vi "teleop2.vi"(7 "Control Type":enum32{"Logitech Joysticks", "Logitech Gamepad"}(ring), 8 "Match Info":T2={"Autonomous Elapsed Seconds"=0.0, "TeleOp Elapsed Seconds"=0.0, "Disabled Elapsed Seconds"=0.0, "Visited Autonomous"=FALSE, "Visited TeleOp"=FALSE, "Visited Disabled"=FALSE, "Autonomous Settings"={"Autonomous Style"=enum."Independent", "VI Refnum"=refnum}}, 11 "Call Context":T1) -> ()   [LabVIEW 2011]
uses:
  <vilib>/Rock Robotics/WPI/DriverStation/WPI_DriverStationMatch Info.ctl
  <vilib>/Rock Robotics/WPI/DriverStation/WPI_DriverStationDerivedRobotMode.ctl
  Robot Global Data.vi
  System Set Points and States.vi
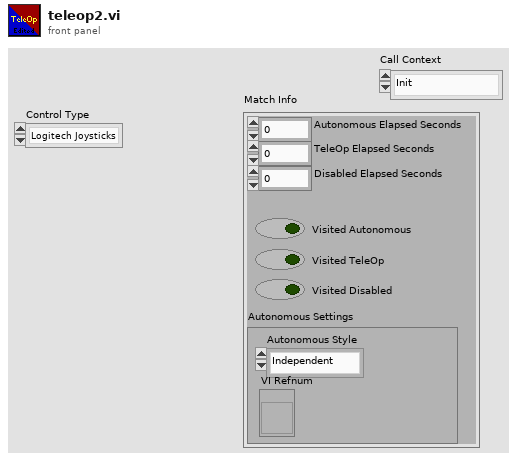
[diagram p1: front panel]
types:
  T1 = typedef "WPI_DriverStationDerivedRobotMode.ctl" = enum16{"Init", "Execute", "Stop"}
  T2 = typedef "WPI_DriverStationMatch Info.ctl" = cluster{"Autonomous Elapsed Seconds":dbl, "TeleOp Elapsed Seconds":dbl, "Disabled Elapsed Seconds":dbl, "Visited Autonomous":bool, "Visited TeleOp":bool, "Visited Disabled":bool, "Autonomous Settings":cluster{"Autonomous Style":enum16{"Iterative", "Independent"}, "VI Refnum":refnum<vi>}}
  T3 = cluster{"Position":cluster{"X":dbl, "Y":dbl}, "Distance (ft)":dbl}[]
  T4 = cluster{"Target Info[0]":cluster{"Position":cluster{"X":dbl, "Y":dbl}, "Distance (ft)":dbl}, "Target Info[1]":cluster{"Position":cluster{"X":dbl, "Y":dbl}, "Distance (ft)":dbl}, "Target Info[2]":cluster{"Position":cluster{"X":dbl, "Y":dbl}, "Distance (ft)":dbl}, "Target Info[3]":cluster{"Position":cluster{"X":dbl, "Y":dbl}, "Distance (ft)":dbl}, "Target Info[4]":cluster{"Position":cluster{"X":dbl, "Y":dbl}, "Distance (ft)":dbl}, "Target Info[5]":cluster{"Position":cluster{"X":dbl, "Y":dbl}, "Distance (ft)":dbl}, "Target Info[6]":cluster{"Position":cluster{"X":dbl, "Y":dbl}, "Distance (ft)":dbl}, "Target Info[7]":cluster{"Position":cluster{"X":dbl, "Y":dbl}, "Distance (ft)":dbl}, "Target Info[8]":cluster{"Position":cluster{"X":dbl, "Y":dbl}, "Distance (ft)":dbl}}
  T5 = typedef "WPI_MotorControlDeviceRef.ctl" = cluster{"DeviceStatus":errorcluster, "Type":enum16{"PWM", "CAN"}, "PWM":cluster{"Digital Module":T6, "PWM Channel":T7, "DeadBand":T8}, "CAN":cluster{"Device Number":u8, "Control Mode":T9, "Semaphore":T10, "Max Vout":dbl}, "Invert":bool, "TransformRef":T11, "InvTransformRef":T11}
  T6 = typedef "FPGA_TypedefDigitalModule.ctl" = enum16{"Digital Module 1", "Digital Module 2"}
  T7 = typedef "FPGA_DIOPWMChannel.ctl" = enum8{"PWM 1", "PWM 2", "PWM 3", "PWM 4", "PWM 5", "PWM 6", "PWM 7", "PWM 8", "PWM 9", "PWM 10", "Invalid"}
  T8 = typedef "WPI_PWMDeadband.ctl" = cluster{"Name":string, "maxPositivePwm":i32, "minPositivePwm":i32, "centerPwm":i32, "maxNegativePwm":i32, "minNegativePwm":i32, "angularRange":u16}
  T9 = typedef "WPI_CANJaguar_ControlMode.ctl" = enum8{"Percent VBus", "Current", "Speed", "Position", "Voltage"}
  T10 = typedef "Semaphore RefNum" = refnum<k1>
  T11 = typedef "WPI_PWMTransform_ConPane.ctl" = refnum<vi>
  T12 = typedef "WPI_JoystickDevRef.ctl" = cluster{"Device":T13}
  T13 = typedef "WPI_JoystickDeviceEnum.ctl" = enum16{"USB 1", "USB 2", "USB 3", "USB 4", "Kinect 1", "Kinect 2"}
  T14 = typedef "WPI_RelayDevRef.ctl" = cluster{"DevStatus":errorcluster, "Relay Channel":T15, "Digital Module":T6, "Relay Direction":T16}
  T15 = typedef "FPGA_DIORelayChannel.ctl" = enum8{"Relay 1", "Relay 2", "Relay 3", "Relay 4", "Relay 5", "Relay 6", "Relay 7", "Relay 8", "Invalid"}
  T16 = typedef "WPI_RelayDirection.ctl" = enum16{"Both directions", "Forward only", "Reverse only"}
  T17 = typedef "WPI_RobotDriveDevRef.ctl" = cluster{"DevStatus":errorcluster, "Motors[]":T5[], "Square Inputs":bool, "Max Output":dbl, "Isochronous":bool}
  T18 = typedef "WPI_JoystickButtonState.ctl" = cluster{"Button 1":bool, "Button 2":bool, "Button 3":bool, "Button 4":bool, "Button 5":bool, "Button 6":bool, "Button 7":bool, "Button 8":bool, "Button 9":bool, "Button 10":bool, "Button 11":bool, "Button 12":bool}
  T19 = cluster{"axis 1 (x)":dbl, "axis 2 (y)":dbl, "axis 3 (throttle)":dbl, "axis 4":dbl, "axis 5":dbl, "axis 6":dbl}
  T20 = typedef "WPI_RelayValue.ctl" = enum16{"Off", "On", "Forward", "Reverse"}
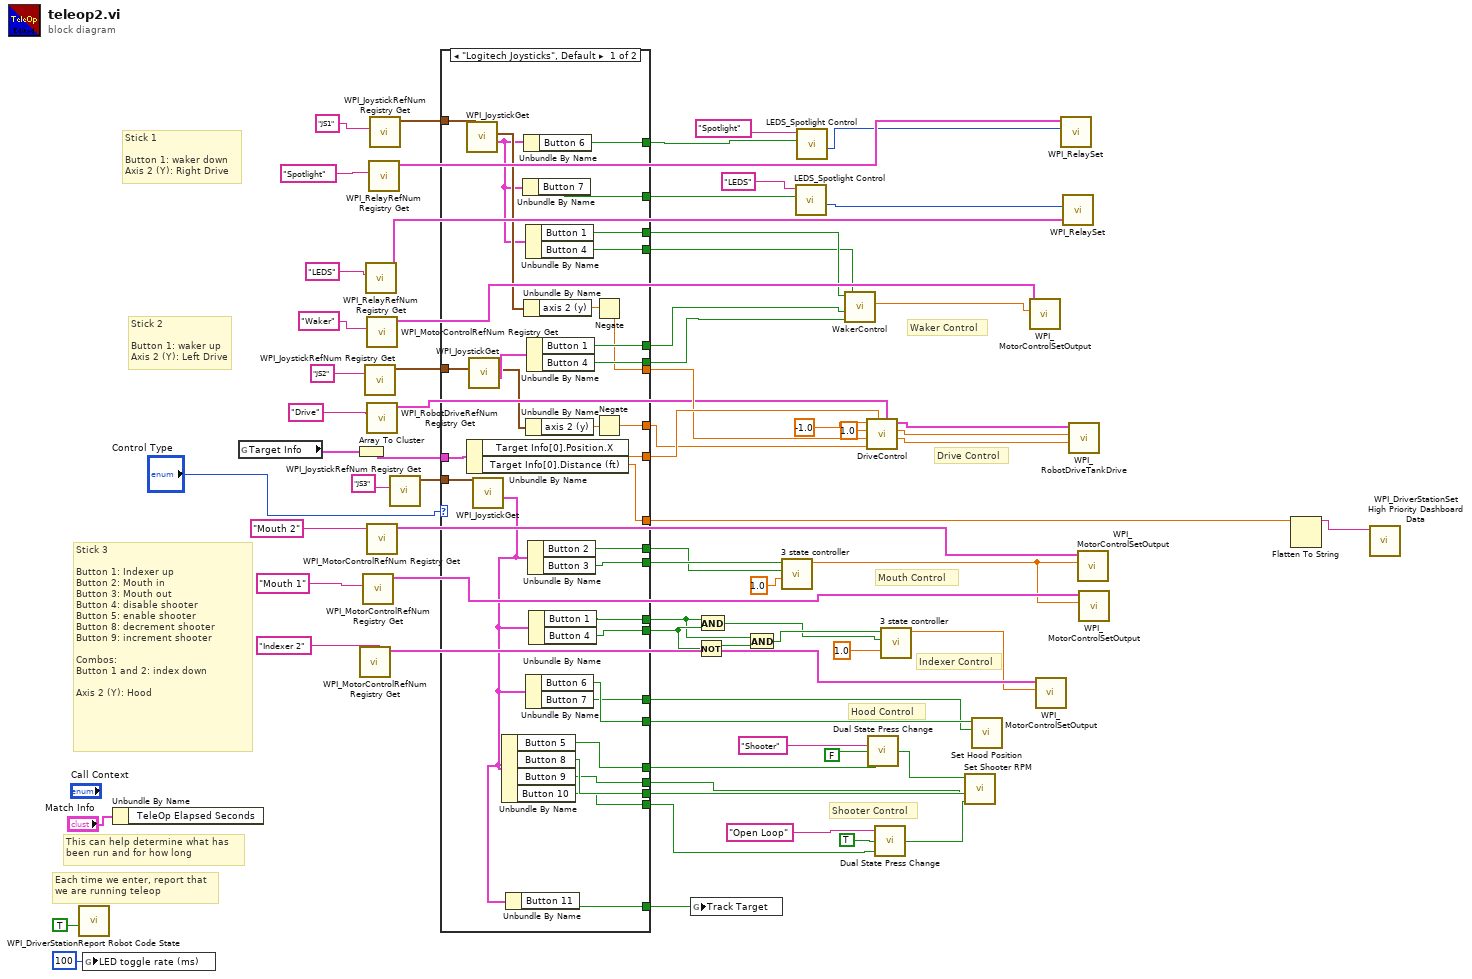
[diagram p0: block diagram]
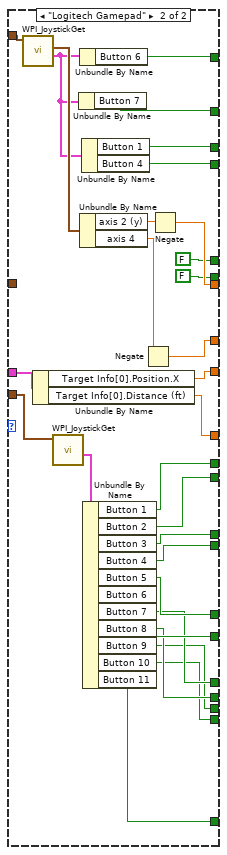
[diagram p2: hidden frame]
diagram:
  # "Each time we enter, report that\nwe are running teleop"
  # "This can help determine what has\nbeen run and for how long"
  # "Drive Control"
  # "Shooter Control"
  # "Hood Control"
  # "Indexer Control"
  # "Stick 3\n\nButton 1: Indexer up\nButton 2: Mouth in\nButton 3: Mouth out\nButton 4: disable shooter\nButton 5: enable shooter\nButton 8: decrement shooter\nButton 9: increment shooter\n\nCombos:\nButton 1 and 2: index down\n \nAxis 2 (Y): Hood"
  # "Stick 2\n\nButton 1: waker up\nAxis 2 (Y): Left Drive"
  # "Stick 1\n\nButton 1: waker down\nAxis 2 (Y): Right Drive"
  # "Waker Control"
  # "Mouth Control"
  n1 = call <vilib>:"WPI_DriverStationReport Robot Code State.vi"("TeleOp"=TRUE ("Autonomous")) -> ()  [unwired: 10 in, 1 out]
  n2 = global write "Robot Global Data.vi" "LED toggle rate (ms)"(u32 100 ("LED ms toggle rate")) -> ()
  n3 = Unbundle By Name("Match Info") -> ()  [unwired: 1 out]
  n4 = global read "Robot Global Data.vi" "Target Info"() -> (w14:T3)
  n5 = Array To Cluster(array=w14) -> (cluster=w13:T4)
  n6 = call <vilib>:"WPI_MotorControlRefNum Registry Get.vi"("refnum name"="Indexer 2") -> ("MotorControlDevRef"=w61:T5)  [unwired: 9 in, 1 out]
  n7 = call <vilib>:"WPI_MotorControlRefNum Registry Get.vi"("refnum name"="Mouth 1") -> ("MotorControlDevRef"=w71:T5)  [unwired: 9 in, 1 out]
  n8 = call <vilib>:"WPI_JoystickRefNum Registry Get.vi"("refnum name"="JS2") -> ("JoystickDevRef"=w11:T12)  [unwired: 9 in, 1 out]
  n9 = call <vilib>:"WPI_RelayRefNum Registry Get.vi"("refnum name"="LEDS") -> ("RelayDevRef"=w59:T14)  [unwired: 9 in, 1 out]
  n10 = call <vilib>:"WPI_MotorControlRefNum Registry Get.vi"("refnum name"="Waker") -> ("MotorControlDevRef"=w60:T5)  [unwired: 9 in, 1 out]
  n11 = call <vilib>:"WPI_RobotDriveRefNum Registry Get.vi"("refnum name"="Drive") -> ("RobotDriveDevRef"=w25:T17)  [unwired: 9 in, 1 out]
  n12 = call <vilib>:"WPI_MotorControlRefNum Registry Get.vi"("refnum name"="Mouth 2") -> ("MotorControlDevRef"=w69:T5)  [unwired: 9 in, 1 out]
  n13 = call <vilib>:"WPI_RelayRefNum Registry Get.vi"("refnum name"="Spotlight") -> ("RelayDevRef"=w65:T14)  [unwired: 9 in, 1 out]
  n14 = call <vilib>:"WPI_JoystickRefNum Registry Get.vi"("refnum name"="JS1") -> ("JoystickDevRef"=w10:T12)  [unwired: 9 in, 1 out]
  n15 = call <vilib>:"WPI_JoystickRefNum Registry Get.vi"("refnum name"="JS3") -> ("JoystickDevRef"=w7:T12)  [unwired: 9 in, 1 out]
  n16 = case shown="\"Logitech Joysticks\", Default" "Control Type" {
    tunnel: [w103 w114] -> w70
    tunnel: [w102 w115] -> w67
    tunnel: [w101 w109] -> w51
    tunnel: [w100 w107] -> w50
    tunnel: [w99 w106] -> w49
    tunnel: [w98 w110] -> w48
    tunnel: [w97 w111] -> w47
    tunnel: [w96 w112] -> w46
    tunnel: [w95 w113] -> w45
    tunnel: [w94 w126] -> w43
    tunnel: [w93 w125] -> w42
    tunnel: [w92 w127] -> w39
    tunnel: [w91 w128] -> w36
    tunnel: [w90 FALSE ("Button 1")] -> w34
    tunnel: [w89 FALSE ("Button 4")] -> w33
    tunnel: [w88 w121] -> w29
    tunnel: [w87 w122] -> w28
    tunnel: [w86 w124] -> w27
    tunnel: [w85 w108] -> w26
    tunnel: [w84 w105] -> w24
    tunnel: w13 -> [w81 w120]
    tunnel: w11 -> [w80 _]
    tunnel: w10 -> [w79 w129]
    tunnel: w7 -> [w75 w117]
    tunnel: [w72 w104] -> w3
    frame "Logitech Joysticks", Default {
      n17 = call <vilib>:"WPI_JoystickGet.vi"("JoystickDevRef"=w79) -> ("Buttons"=w74:T18, "Axes"=w76:T19)  [unwired: 4 in, 1 out]
      n18 = Unbundle By Name(w81) -> ("Target Info[0].Position.X"=w88:dbl, "Target Info[0].Distance (ft)"=w72:dbl)
      n19 = call <vilib>:"WPI_JoystickGet.vi"("JoystickDevRef"=w80) -> ("Buttons"=w78:T18, "Axes"=w77:T19)  [unwired: 4 in, 1 out]
      n20 = call <vilib>:"WPI_JoystickGet.vi"("JoystickDevRef"=w75) -> ("Buttons"=w73:T18)  [unwired: 4 in, 2 out]
      n21 = Unbundle By Name(w73) -> ("Button 5"=w101:bool, "Button 8"=w100:bool, "Button 9"=w85:bool, "Button 10"=w99:bool)
      n22 = Unbundle By Name(w73) -> ("Button 11"=w84:bool)
      n23 = Unbundle By Name(w74) -> ("Button 7"=w92:bool)
      n24 = Unbundle By Name(w74) -> ("Button 6"=w91:bool)
      n25 = Unbundle By Name(w76) -> ("axis 2 (y)"=w82:dbl)
      n26 = Unbundle By Name(w74) -> ("Button 1"=w94:bool, "Button 4"=w93:bool)
      n27 = Unbundle By Name(w77) -> ("axis 2 (y)"=w83:dbl)
      n28 = Unbundle By Name(w73) -> ("Button 6"=w98:bool, "Button 7"=w97:bool)
      n29 = Unbundle By Name(w78) -> ("Button 1"=w90:bool, "Button 4"=w89:bool)
      n30 = Unbundle By Name(w73) -> ("Button 2"=w102:bool, "Button 3"=w103:bool)
      n31 = Unbundle By Name(w73) -> ("Button 1"=w95:bool, "Button 4"=w96:bool)
      n32 = Negate(x=w82) -> (-x=w86:dbl)
      n33 = Negate(x=w83) -> (-x=w87:dbl)
    }
    frame "Logitech Gamepad" {
      n34 = call <vilib>:"WPI_JoystickGet.vi"("JoystickDevRef"=w129) -> ("Buttons"=w130:T18, "Axes"=w131:T19)  [unwired: 4 in, 1 out]
      n35 = Unbundle By Name(w120) -> ("Target Info[0].Position.X"=w121:dbl, "Target Info[0].Distance (ft)"=w104:dbl)
      n36 = call <vilib>:"WPI_JoystickGet.vi"("JoystickDevRef"=w117) -> ("Buttons"=w116:T18)  [unwired: 4 in, 2 out]
      n37 = Unbundle By Name(w130) -> ("Button 7"=w127:bool)
      n38 = Unbundle By Name(w130) -> ("Button 6"=w128:bool)
      n39 = Unbundle By Name(w131) -> ("axis 2 (y)"=w132:dbl, "axis 4"=w123:dbl)
      n40 = Unbundle By Name(w130) -> ("Button 1"=w126:bool, "Button 4"=w125:bool)
      n41 = Unbundle By Name(w116) -> ("Button 1"=w115:bool, "Button 2"=w114:bool, "Button 3"=w113:bool, "Button 4"=w112:bool, "Button 5"=w111:bool, "Button 6"=w110:bool, "Button 7"=w109:bool, "Button 8"=w108:bool, "Button 9"=w107:bool, "Button 10"=w106:bool, "Button 11"=w105:bool)
      n42 = Negate(x=w123) -> (-x=w122:dbl)
      n43 = Negate(x=w132) -> (-x=w124:dbl)
    }
  }
  n44 = global write "System Set Points and States.vi" "Track Target"(w24) -> ()
  n45 = Not(x=w46) -> (.not. x?=w52:bool)
  n46 = And(x=w45, y=w46) -> (x .and. y?=w63:bool)
  n47 = And(x=w45, y=w52) -> (x .and. y?=w64:bool)
  n48 = call "3 state controller.vi"("Power"=1.0, "Backward"=w67, "Forward"=w70) -> ("Numeric"=w68:dbl)  [unwired: 8 in]
  n49 = call "LEDS_Spotlight Control.vi"("LEDs or Spotlight"="LEDS", "JS 1 Button 7"=w39) -> ("Relay State"=w40:T20)  [unwired: 8 in]
  n50 = call "LEDS_Spotlight Control.vi"("LEDs or Spotlight"="Spotlight", "JS 1 Button 7"=w36) -> ("Relay State"=w35:T20)  [unwired: 8 in]
  n51 = call "WakerControl.vi"("JS2 Button 4"=w33, "JS2 Button 1"=w34, "JS1 Button 4"=w42, "JS1 Button 1"=w43) -> ("Speed Out"=w41:dbl)  [unwired: 5 in]
  n52 = call "DriveControl.vi"("RobotDriveDevRef"=w25, "Xvalue of Target"=w29, "Right axis value"=w28, "Left axis value"=w27, "Lower Bound"=1.0, "Upper Bound"=-1.0) -> ("Set Right Speed"=w30:dbl, "Set Left Speed"=w31:dbl, "RobotDriveDevRef"=w32:T17)  [unwired: 3 in]
  n53 = call "Dual State Press Change.vi"("Enable/Disable"=w51, "Initial"=FALSE, "Value Name"="Shooter") -> ("Enabled"=w56:bool)
  n54 = call "Dual State Press Change.vi"("Enable/Disable"=w49, "Initial"=TRUE, "Value Name"="Open Loop") -> ("Enabled"=w53:bool)
  n55 = call "3 state controller.vi"("Power"=1.0, "Backward"=w63, "Forward"=w64) -> ("Numeric"=w44:dbl)  [unwired: 8 in]
  n56 = call "Set Shooter RPM.vi"("Open Loop"=w53, "Increment"=w26, "Decrement"=w50, "Shooter Enabled"=w56) -> ()  [unwired: 8 in]
  n57 = call "Set Hood Position.vi"("Increment"=w47, "Decrement"=w48) -> ()  [unwired: 10 in]
  n58 = call <vilib>:"WPI_MotorControlSetOutput.vi"("Output"=w41, "MotorControlDevRef"=w60) -> ()  [unwired: 8 in, 2 out]
  n59 = call <vilib>:"WPI_MotorControlSetOutput.vi"("Output"=w44, "MotorControlDevRef"=w61) -> ()  [unwired: 8 in, 2 out]
  n60 = call <vilib>:"WPI_RelaySet.vi"("RelayValue"=w35, "RelayDevRef"=w65) -> ()  [unwired: 8 in, 2 out]
  n61 = call <vilib>:"WPI_RelaySet.vi"("RelayValue"=w40, "RelayDevRef"=w59) -> ()  [unwired: 8 in, 2 out]
  n62 = call <vilib>:"WPI_RobotDriveTankDrive.vi"("Right axis value"=w30, "Left axis value"=w31, "RobotDriveDevRef"=w32) -> ()  [unwired: 7 in, 2 out]
  n63 = call <vilib>:"WPI_MotorControlSetOutput.vi"("Output"=w68, "MotorControlDevRef"=w69) -> ()  [unwired: 8 in, 2 out]
  n64 = call <vilib>:"WPI_MotorControlSetOutput.vi"("Output"=w68, "MotorControlDevRef"=w71) -> ()  [unwired: 8 in, 2 out]
  n65 = Flatten To String(anything=w3) -> (data string=w4:string)  [unwired: 3 in, 2 out]
  n66 = call <vilib>:"WPI_DriverStationSet High Priority Dashboard Data.vi"("User Data"=w4) -> ()  [unwired: 10 in, 1 out]
